vi "vers_19.vi"() -> ()   [LabVIEW 2019]
uses:
  <vilib>/numeric/Random Number (Range) U64.vi
  <vilib>/numeric/Random Number (Range) I64.vi
panel:
  in  "Stop":bool
  in  "milisecond to wait":dbl
  out "x,y":dbl
  in  "Stop Button 2":bool
  out "String":string
  out "Yinelenen X,Y":dbl[](array[numeric])
  out "X,Y":dbl[](array[numeric])
  out "Tekrarlı index\nnumara saysı":i32
  out "Kalan İndex sayısı":i32
  out "Boolean":bool
  out "Eklenen Sayı":dbl format="%#.1f"
  in  "Rastgele_Doldur":bool
  in  "0'la Doldur":bool
  out "Array":i32[][](array[numeric])
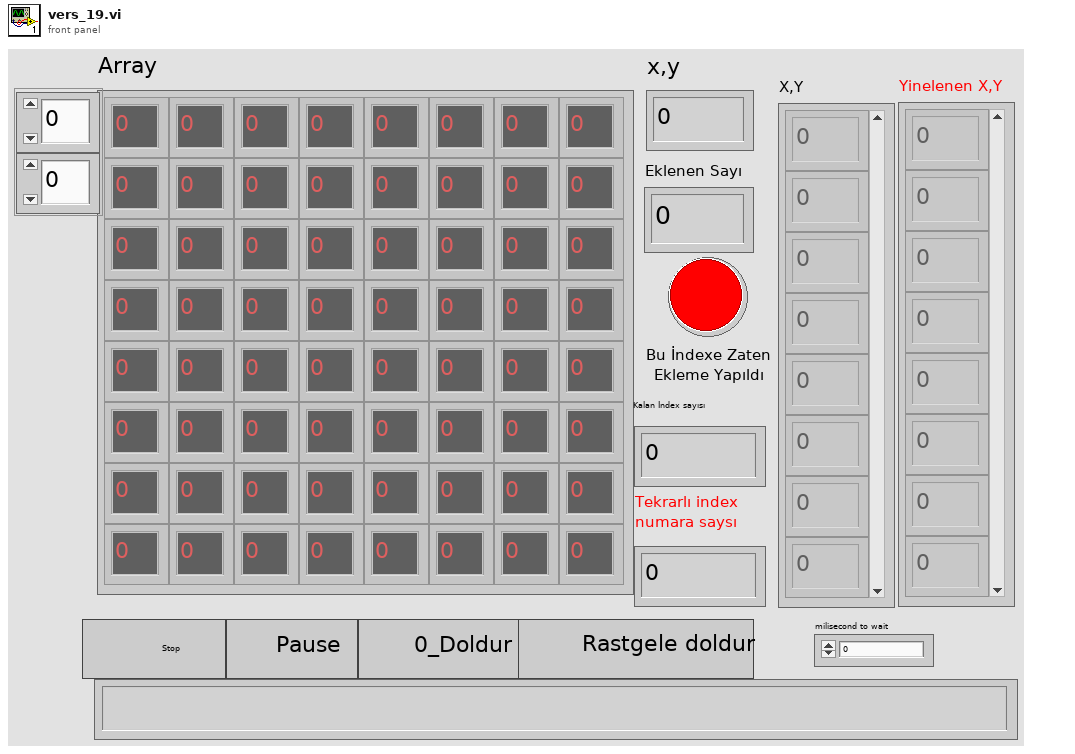
[diagram p1: front panel]
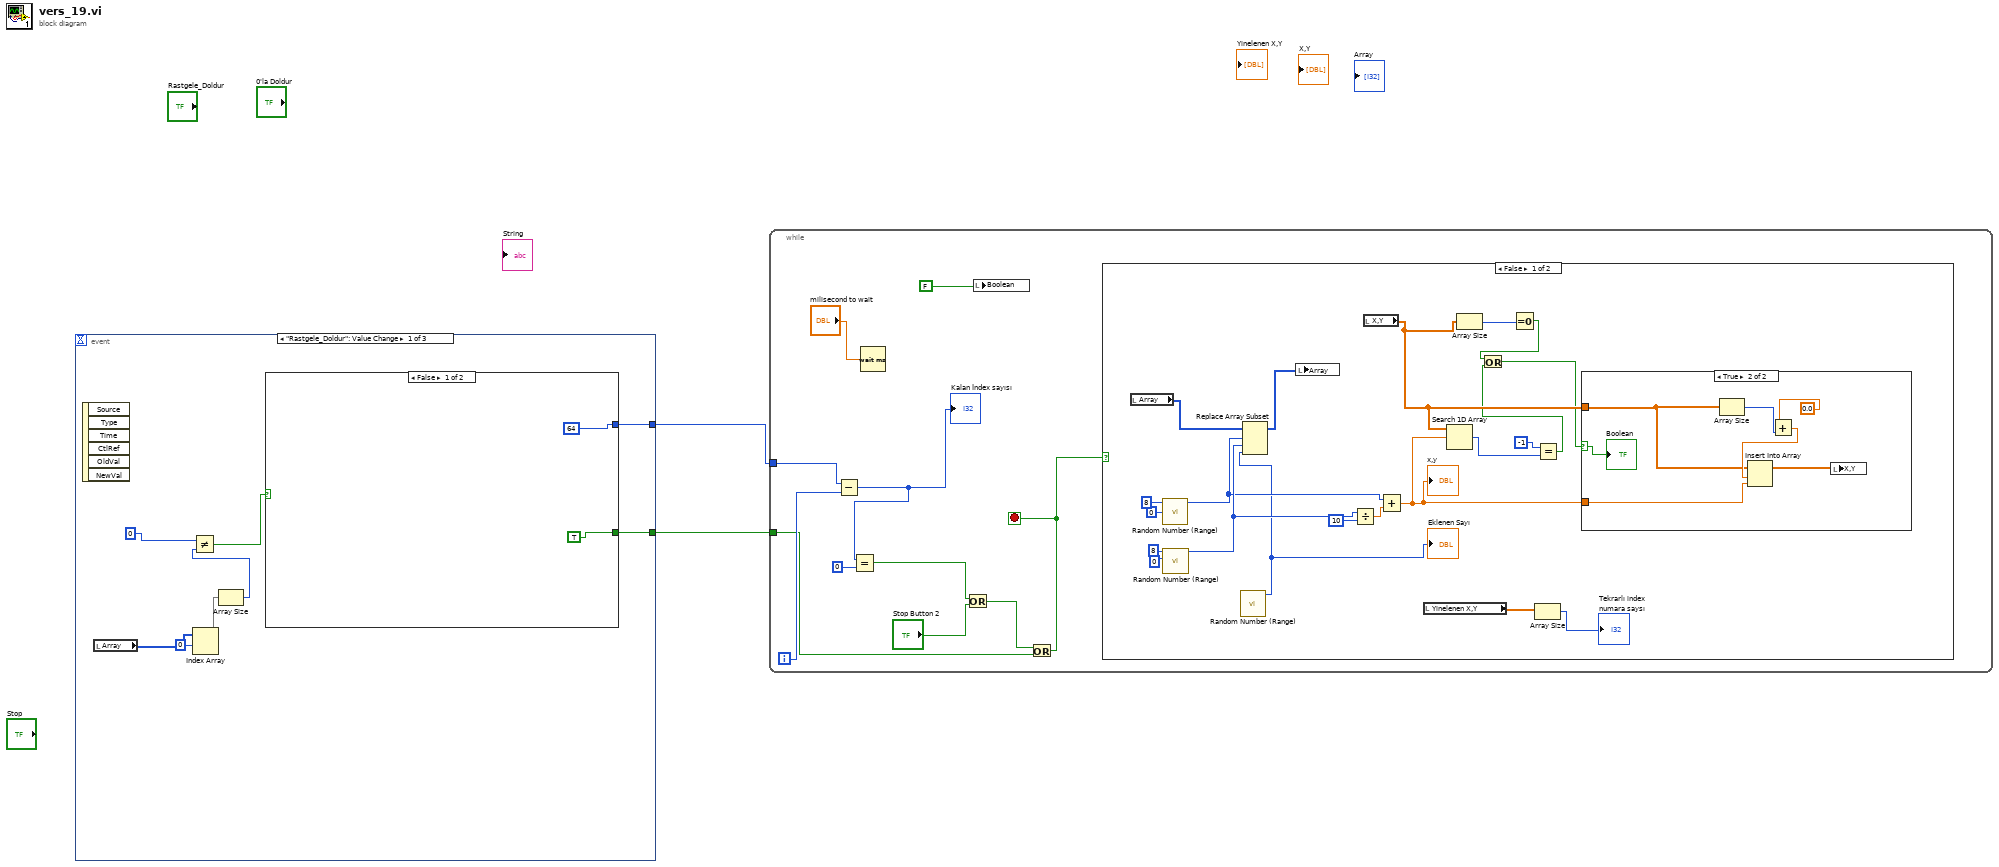
[diagram p0: block diagram]
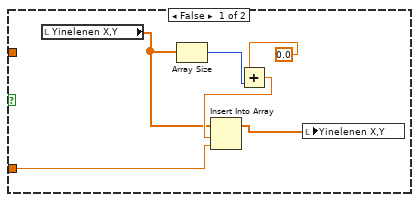
[diagram p2: hidden frame]
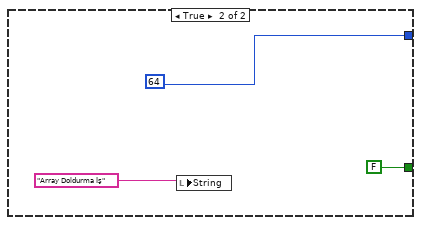
[diagram p4: hidden frame]
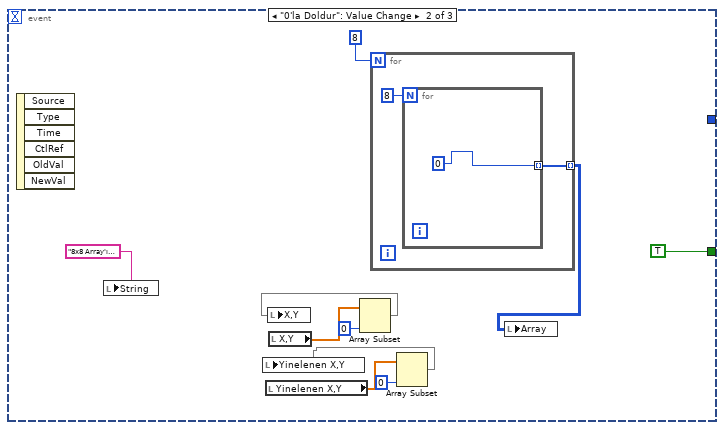
[diagram p5: hidden frame]
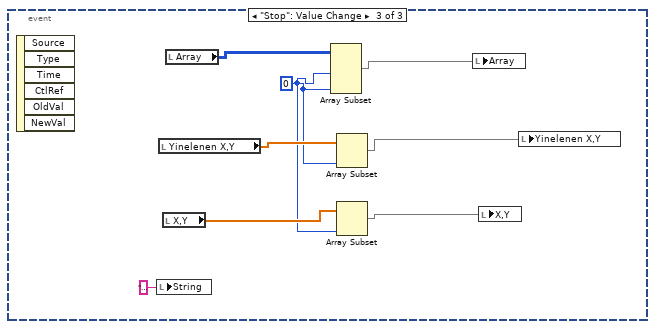
[diagram p6: hidden frame]
diagram:
  n1 = event shown="[0] \"Rastgele_Doldur\": Value Change" {
    selector: _ -> [_ _ _]
    dyn-events: _ -> [_ _ _]
    timeout: _ -> [_ _ _]
    tunnel: [w9 _ _] -> w2
    tunnel: [w10 TRUE _] -> w1
    event "Rastgele_Doldur": Value Change {
      n2 = event-data() -> ()  [unwired: 1 in, 6 out]
      n3 = local read "Array"() -> (w7:i32[][])
      n4 = Index Array(array=w7, index (row)=0) -> (element=w5:i32[])  [unwired: 1 in]
      n5 = Array Size(array=w5) -> (size(s)=w4:i32)
      n6 = Not Equal?(x=0 ("size(s)"), y=w4) -> (x != y?=w3:bool)
      n7 = case shown="False" w3 {
        tunnel: [TRUE FALSE] -> w10
        tunnel: [64 64] -> w9
        frame False {
        }
        frame True {
          n8 = local write "String"("Array Doldurma İş") -> ()
        }
      }
    }
    event "0'la Doldur": Value Change {
      n9 = event-data() -> ()  [unwired: 1 in, 6 out]
      n10 = local write "String"("8x8 Array'ı 0'la Dolduruldu. Şimdi \"Rastgele Doldur\" Butonuna Basabilirsiniz") -> ()
      n11 = local read "Yinelenen X,Y"() -> (w25:dbl[])
      n12 = local read "X,Y"() -> (w23:dbl[])
      n13 = Array Subset(array=w23, length=0) -> (w22:dbl[])  [unwired: 1 in]
      n14 = local write "X,Y"(w22) -> ()
      n15 = for {
        N: 8 -> [_]
        tunnel: [w26] -> w17 mode=indexing
        n16 = for {
          N: 8 -> [_]
          tunnel: [0] -> w26 mode=indexing
        }
      }
      n17 = Array Subset(array=w25, length=0) -> (w24:dbl[])  [unwired: 1 in]
      n18 = local write "Yinelenen X,Y"(w24) -> ()
      n19 = local write "Array"(w17) -> ()
    }
    event "Stop": Value Change {
      w29 = 0
      n20 = event-data() -> ()  [unwired: 1 in, 6 out]
      n21 = local write "String"("ı 0'la Dolduruldu. Şimdi \"Rastgele Doldur\" Butonuna Basabilirsiniz" ("String")) -> ()
      n22 = local read "Yinelenen X,Y"() -> (w34:dbl[])
      n23 = local read "X,Y"() -> (w36:dbl[])
      n24 = local read "Array"() -> (w32:i32[][])
      n25 = Array Subset(array=w32, length (row)=w29, length (col)=w29) -> (w31:i32[][])  [unwired: 2 in]
      n26 = Array Subset(array=w34, length=w29) -> (w33:dbl[])  [unwired: 1 in]
      n27 = Array Subset(array=w36, length=w29) -> (w35:dbl[])  [unwired: 1 in]
      n28 = local write "Array"(w31) -> ()
      n29 = local write "X,Y"(w35) -> ()
      n30 = local write "Yinelenen X,Y"(w33) -> ()
    }
  }
  n31 = while {
    tunnel: w2 -> [w46]
    tunnel: w1 -> [w39]
    i -> [w47]
    stop <- w38 stop-if-true
    n32 = Subtract(x=w46, y=w47) -> (x-y=w45:i32)
    "Kalan İndex sayısı" <- w45
    n33 = Equal?(x=w45, y=u64 0) -> (x = y?=w43:bool)
    n34 = Wait (ms)(milliseconds to wait="milisecond to wait") -> ()  [unwired: 1 out]
    n35 = Or(x=w43, y="Stop Button 2") -> (x .or. y?=w40:bool)
    n36 = local write "Boolean"(FALSE) -> ()
    n37 = Or(x=w40, y=w39) -> (x .or. y?=w38:bool)
    n38 = case shown="False" w38 {
      frame False {
        n39 = local read "Array"() -> (w48:i32[][])
        n40 = call-poly <vilib>:"Random Number (Range).vi"("lower bound (-100)"=0, "upper bound (100)"=8) -> ("number"=w61:i64)  [unwired: 9 in]
        n41 = call-poly <vilib>:"Random Number (Range).vi"("lower bound (-100)"=0, "upper bound (100)"=8) -> ("number"=w64:i64)  [unwired: 9 in]
        n42 = call-poly <vilib>:"Random Number (Range).vi"() -> ("number"=w60:u64)  [unwired: 11 in]
        "Eklenen Sayı" <- w60
        n43 = Replace Array Subset(array=w48, new element=w60, index (row)=w61, index (col)=w64) -> (w49:i32[][])
        n44 = local write "Array"(w49) -> ()
        n45 = Divide(x=w64, y=i64 10) -> (x/y=w62:dbl)
        n46 = local read "X,Y"() -> (w52:dbl[])
        n47 = Add(x=w61, y=w62) -> (x+y=w57:dbl)
        "x,y" <- w57
        n48 = local read "Yinelenen X,Y"() -> (w56:dbl[])
        n49 = Search 1D Array(1D array=w52, element=w57) -> (index of element=w59:i32)  [unwired: 1 in]
        n50 = Array Size(array=w52) -> (size(s)=w54:i32)
        n51 = Equal To 0?(x=w54) -> (x = 0?=w53:bool)
        n52 = Array Size(array=w56) -> (size(s)=→"Tekrarlı index\nnumara saysı":i32)
        n53 = Equal?(x=-1, y=w59) -> (x = y?=w51:bool)
        n54 = Or(x=w53, y=w51) -> (x .or. y?=w50:bool)
        n55 = case shown="True" w50 {
          selector: w50 -> [_ w75]
          tunnel: w52 -> [_ w77]
          tunnel: w57 -> [w71 w76]
          frame False {
            n56 = local read "Yinelenen X,Y"() -> (w69:dbl[])
            n57 = Array Size(array=w69) -> (size(s)=w73:i32)
            n58 = Add(x=0.0, y=w73) -> (x+y=w74:dbl)
            n59 = Insert Into Array(array=w69, index=w74, new element=w71) -> (w70:dbl[])
            n60 = local write "Yinelenen X,Y"(w70) -> ()
          }
          frame True {
            n61 = Array Size(array=w77) -> (size(s)=w80:i32)
            n62 = Add(x=0.0, y=w80) -> (x+y=w81:dbl)
            n63 = Insert Into Array(array=w77, index=w81, new element=w76) -> (w79:dbl[])
            n64 = local write "X,Y"(w79) -> ()
            "Boolean" <- w75
          }
        }
      }
      frame True {
      }
    }
  }
